vi "Login.vi"(9 "error in":errorcluster, 10 "产品型号":refnum<vi>) -> (1 "error out":errorcluster, 2 "Access":bool)   [LabVIEW 2013]
doc: "This VI is the solution to Exercise 3-1 of the LabVIEW Basics II course.\n\nThis VI will accept a user name and password, and after the OK button is pressed, verify if the information is valid using the Verify Information subVI. The name and password controls are initialized to empty strings and the Key Focus attribute of the Login Name control is set to TRUE.\n\nYou will use this VI in Application Exercise.vi (Exercise 5-1) as your login screen."
uses:
  GlobValue.vi
  <vilib>/Utility/config.llb/Read Key (String).vi
  <vilib>/Utility/config.llb/NI_LVConfig.lvlib
panel:
  out "User":string caption="值"
  out "ps":string caption="值"
  in  "Cancle":bool
  in  "Ok":bool
  in  "Password":string
  in  "Login Name":string
  # "用户登录"
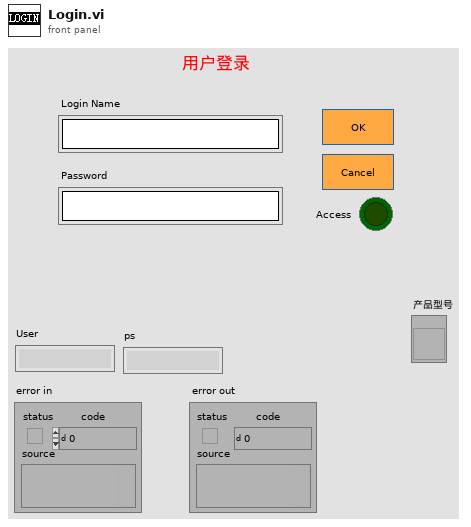
[diagram p1: front panel]
types:
  T1 = typedef "NI_LVConfig.lvlib/Config Data RefNum.ctl" = refnum<k1>
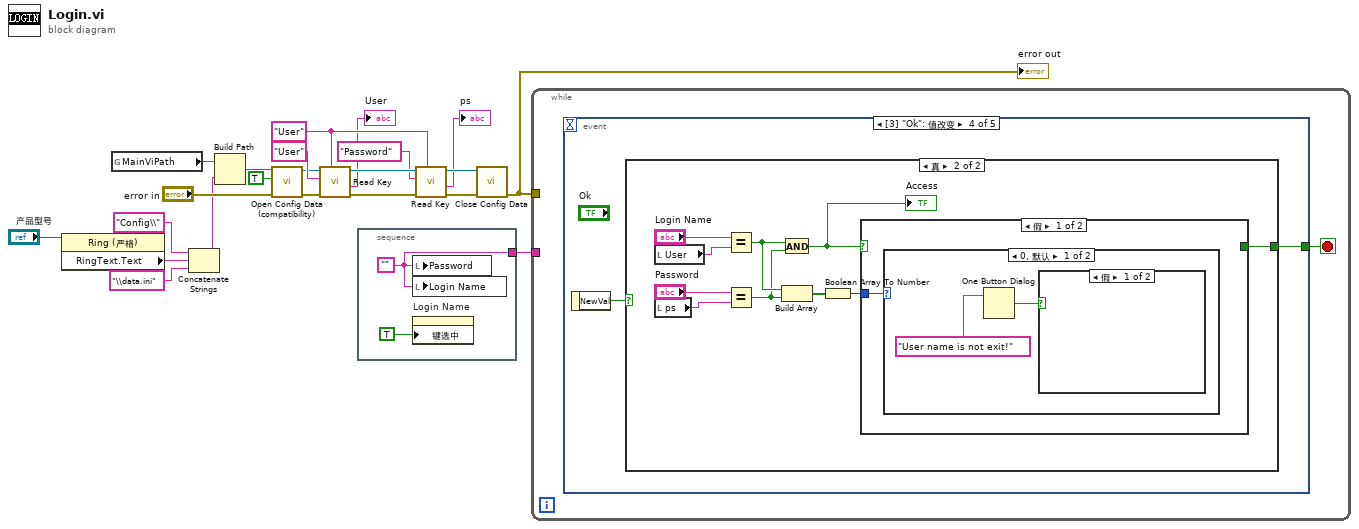
[diagram p0: block diagram]
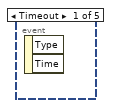
[diagram p2: hidden frame]
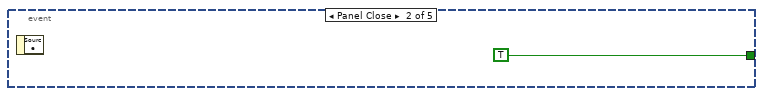
[diagram p3: hidden frame]
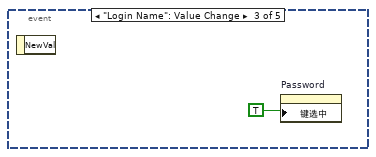
[diagram p4: hidden frame]
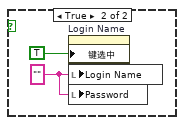
[diagram p6: hidden frame]
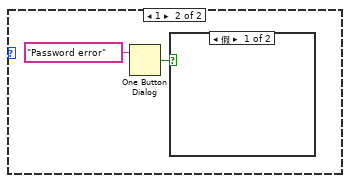
[diagram p7: hidden frame]
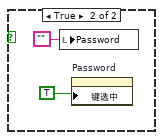
[diagram p8: hidden frame]
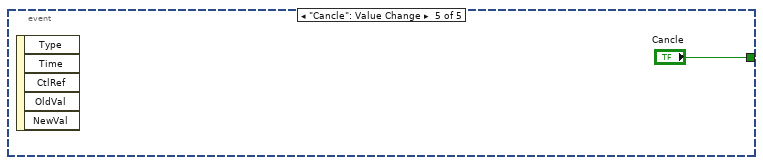
[diagram p10: hidden frame]
diagram:
  w16 = "User" ("ModelName")
  n1 = property class="Ring (严格)"(reference="产品型号") -> ("RingText.Text"=w3:string)  [unwired: 1 in, 2 out]
  n2 = global read "GlobValue.vi" "MainViPath"() -> (w7:path)
  n3 = Concatenate Strings("Config\\" ("名称或相对路径"), w3, "\\data.ini") -> (w1:string)
  n4 = Build Path(base path=w7, name or relative path=w1) -> (appended path=w20:path)
  n5 = call <vilib>:"Open Config Data (compatibility).vi"("error in (no error)"="error in", "create file if necessary (T)"=TRUE, "configuration file path"=w20) -> ("error out"=w12:errorcluster, "refnum"=w14:T1)  [unwired: 6 in, 1 out]
  n6 = call-poly <vilib>:"Read Key.vi"("section"=w16, "error in (no error)"=w12, "key"="User", "refnum"=w14) -> ("error out"=w17:errorcluster, "value"=→"User":string, "refnum out"=w18:T1)  [unwired: 2 in, 3 out]
  n7 = stacked-sequence {
    tunnel: [w23] -> w22
    frame #0 {
      w23 = ""
      n8 = local write "Password"(w23) -> ()
      n9 = local write "Login Name"(w23) -> ()
      n10 = property on="Login Name" class="Str"("键选中"=TRUE ("Key Focus")) -> ()  [unwired: 2 in, 2 out]
    }
  }
  n11 = call-poly <vilib>:"Read Key.vi"("section"=w16, "error in (no error)"=w17, "key"="Password", "refnum"=w18) -> ("error out"=w8:errorcluster, "value"=→"ps":string, "refnum out"=w13:T1)  [unwired: 2 in, 3 out]
  n12 = call <vilib>:"Close Config Data.vi"("error in (no error)"=w8, "refnum"=w13) -> ("error out"=w6:errorcluster)  [unwired: 1 in, 8 out]
  "error out" <- w6
  n13 = while {
    tunnel: w22 -> [_]
    tunnel: w6 -> [_]
    stop <- w25 stop-if-true
    n14 = event shown="[3] \"Ok\": 值改变" {
      selector: _ -> [_ _ _ _ _]
      dyn-events: _ -> [_ _ _ _ _]
      timeout: _ -> [_ _ _ _ _]
      tunnel: [_ TRUE ("Cancle") _ w28 "Cancle"] -> w25
      event Timeout {
        n15 = event-data() -> ()  [unwired: 3 out]
      }
      event Panel Close {
        n16 = event-data() -> ()  [unwired: 2 out]
      }
      event "Login Name": Value Change {
        n17 = event-data() -> ()  [unwired: 2 out]
        n18 = property on="Password" class="Str"("键选中"=TRUE ("Key Focus")) -> ()  [unwired: 2 in, 2 out]
      }
      event "Ok": Value Change {
        n19 = event-data() -> ("NewVal"=w29:bool)  [unwired: 1 out]
        n20 = case shown="真" w29 {
          tunnel: [_ w39] -> w28
          frame False {
          }
          frame True {
            n21 = local read "User"() -> (w35:string)
            n22 = local read "ps"() -> (w36:string)
            n23 = Equal?(x="Login Name", y=w35) -> (x = y?=w33:bool)
            n24 = Equal?(x="Password", y=w36) -> (x = y?=w32:bool)
            n25 = And(x=w33, y=w32) -> (x .and. y?=w34:bool)
            "Access" <- w34
            n26 = Build Array(w33, w32) -> (w31:bool[])
            n27 = Boolean Array To Number(Boolean array=w31) -> (number=w30:u32)
            n28 = case shown="假" w34 {
              selector: w34 -> [_ w49]
              tunnel: [_ w49] -> w39
              tunnel: w30 -> [w40 _]
              frame False {
                n29 = case shown="0, 默认" w40 {
                  frame 0, Default {
                    n30 = One Button Dialog(message="User name is not exit!" ("消息")) -> (true=w41:bool)  [unwired: 1 out]
                    n31 = case shown="假" w41 {
                      frame False {
                      }
                      frame True {
                        w43 = "" ("Login Name")
                        n32 = property on="Login Name" class="Str"("键选中"=TRUE ("Key Focus")) -> ()  [unwired: 2 in, 2 out]
                        n33 = local write "Login Name"(w43) -> ()
                        n34 = local write "Password"(w43) -> ()
                      }
                    }
                  }
                  frame 1 {
                    n35 = One Button Dialog(message="Password error" ("消息")) -> (true=w45:bool)  [unwired: 1 out]
                    n36 = case shown="假" w45 {
                      frame False {
                      }
                      frame True {
                        n37 = local write "Password"("") -> ()
                        n38 = property on="Password" class="Str"("键选中"=TRUE ("Key Focus")) -> ()  [unwired: 2 in, 2 out]
                      }
                    }
                  }
                }
              }
              frame True {
              }
            }
          }
        }
      }
      event "Cancle": Value Change {
        n39 = event-data() -> ()  [unwired: 6 out]
      }
    }
  }
